vi "Test_Valco_Valve.vi"() -> ()   [LabVIEW 2011]
uses:
  ADAM Client/Sub VIs/ADAM Controls/Valco_valve_ph.ctl
panel:
  in  "stop":bool
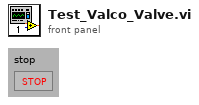
[diagram p1: front panel]
types:
  T1 = typedef "Valco_valve_ph.ctl" = u16
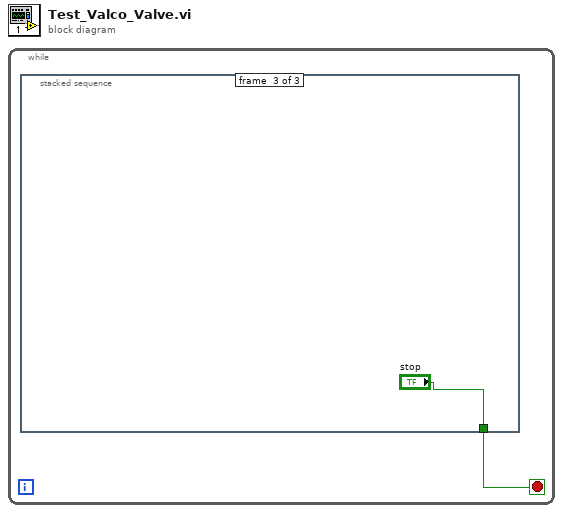
[diagram p0: block diagram]
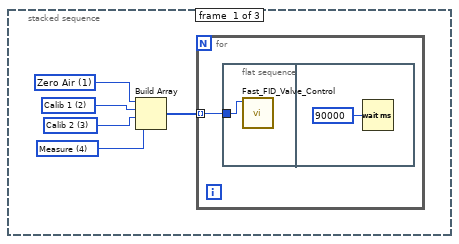
[diagram p2: hidden frame]
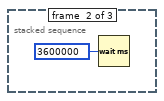
[diagram p3: hidden frame]
diagram:
  n1 = while {
    stop <- w1 stop-if-true
    n2 = stacked-sequence {
      tunnel: [_ _ "stop"] -> w1
      frame #0 {
        w3 = T1 4 items=["", "Zero Air", "Calib 1", "Calib 2", "Measure"] ("Requested Position")
        w4 = T1 3 items=["", "Zero Air", "Calib 1", "Calib 2", "Measure"] ("Requested Position")
        w5 = T1 2 items=["", "Zero Air", "Calib 1", "Calib 2", "Measure"] ("Requested Position")
        w6 = T1 1 items=["", "Zero Air", "Calib 1", "Calib 2", "Measure"] ("Requested Position")
        n3 = Build Array(w6, w5, w4, w3) -> (w2:T1[])
        n4 = for {
          tunnel: w2 -> [w7] mode=indexing
          n5 = flat-sequence {
            tunnel: w7 -> [w8]
            frame #0 {
              n6 = call "Fast_FID_Valve_Control.vi"("Requested Position"=w8) -> ()  [unwired: 5 in, 2 out]
            }
            frame #1 {
              n7 = Wait (ms)(milliseconds to wait=u32 90000) -> ()  [unwired: 1 out]
            }
          }
        }
      }
      frame #1 {
        n8 = Wait (ms)(milliseconds to wait=u32 3600000) -> ()  [unwired: 1 out]
      }
      frame #2 {
      }
    }
  }
